vi "LHF.DB.Mongo.Collection.FindAndModify.vi"(6 "fields":refnum<k24>, 8 "error in (no error)":errorcluster, 9 "query":refnum<k24>, 10 "Collection":string, 11 "LHF.DB.Mongo in":refnum<class "LHF.DB.Mongo.lvclass">) -> (0 "error out":errorcluster, 2 "Document":string, 3 "LHF.DB.Mongo out":refnum<class "LHF.DB.Mongo.lvclass">, 5 "_id":string)   [LabVIEW 2013]
uses:
  LHF.DB.Mongo.lvclass
  C:/Users/Ricardo/Desktop/Projetos/LabVIEW-MongoDB/src/Driver/MongoDB.Driver.dll
  Driver/MongoDB.Driver.dll
  C:/Users/Ricardo/Desktop/Projetos/LabVIEW-MongoDB/src/Driver/MongoDB.Bson.dll
  Driver/MongoDB.Bson.dll
panel:
  in  "update":refnum<k24>
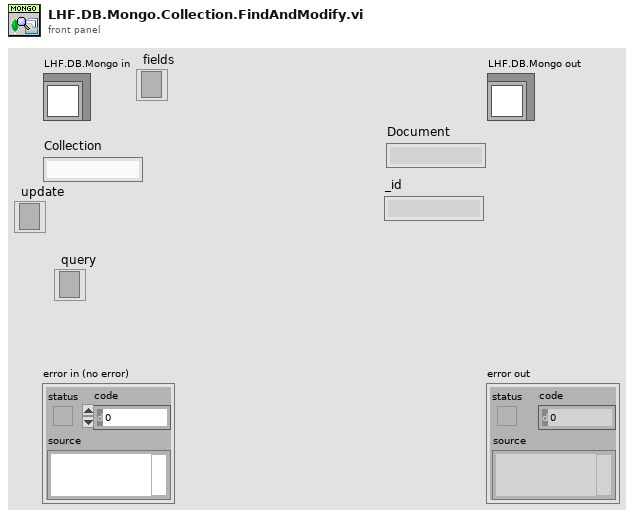
[diagram p1: front panel]
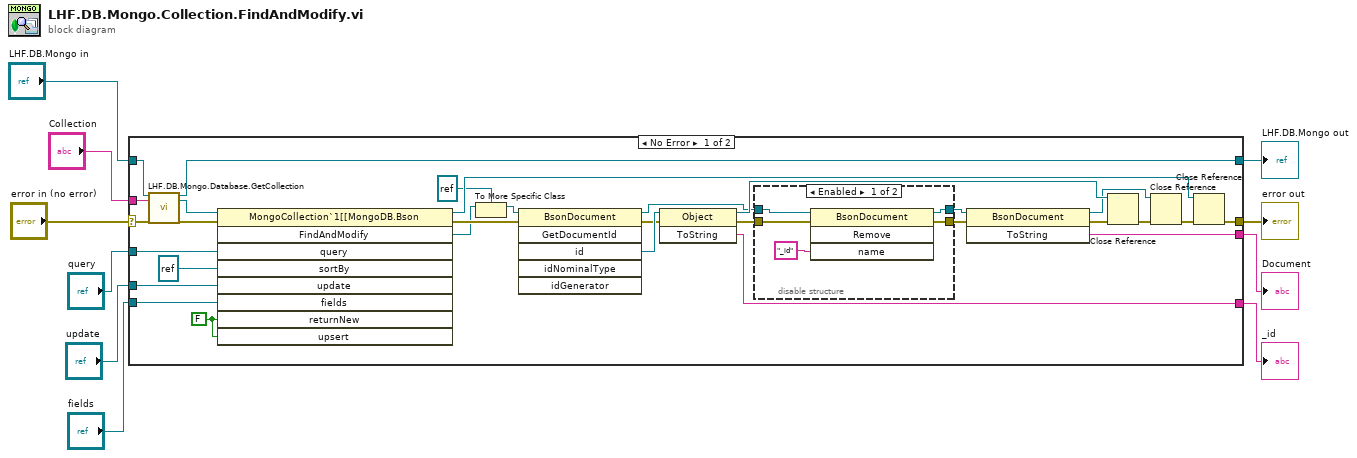
[diagram p0: block diagram]
diagram:
  n1 = case shown="No Error" "error in (no error)" {
    selector: "error in (no error)" -> [w34 w49]
    tunnel: [w36 w49] -> w9
    tunnel: [w39 w48] -> w7
    tunnel: "LHF.DB.Mongo in" -> [w38 w48]
    tunnel: "Collection" -> [w40 _]
    tunnel: "query" -> [w19 _]
    tunnel: [w21 _] -> w4
    tunnel: [w20 _] -> w3
    tunnel: "fields" -> [w12 _]
    tunnel: "update" -> [w11 _]
    frame No Error {
      w13 = FALSE ("returnNew")
      n2 = call "LHF.DB.Mongo.Database.GetCollection.vi"("LHF.DB.Mongo in"=w38, "collectionName"=w40, "error in (no error)"=w34) -> ("LHF.DB.Mongo in"=w39:refnum<class "LHF.DB.Mongo.lvclass">, "MongoCollection"=w35:refnum<k24>, "error out"=w33:errorcluster)  [unwired: 14 in]
      n3 = invoke class="MongoCollection`1[[MongoDB.Bson" method="FindAndModify"(reference=w35, error in=w33, "query"=w19, "sortBy"=refnum<k24> refnum, "update"=w11, "fields"=w12, "returnNew"=w13, "upsert"=w13) -> (reference out=w37:refnum<k24>, error out=w18:errorcluster, "FindAndModify"=w17:refnum<k24>)  [unwired: 1 in, 6 out]
      n4 = To More Specific Class(target class=refnum<k24> refnum ("BsonDocument"), reference=w17) -> (specific class reference=w16:refnum<k24>)  [unwired: 1 in, 1 out]
      n5 = invoke class="BsonDocument" method="GetDocumentId"(reference=w16, error in=w18) -> (reference out=w26:refnum<k24>, error out=w31:errorcluster, "id"=w32:refnum<k24>)  [unwired: 4 in, 3 out]
      n6 = invoke class="Object" method="ToString"(reference=w32, error in=w31) -> (reference out=w29:refnum<k24>, error out=w27:errorcluster, "ToString"=w21:string)  [unwired: 1 in]
      n7 = disable-structure shown="Enabled" {
        disable-tunnel: [w44 w47] -> w28
        disable-tunnel: w27 -> [w43 w46]
        disable-tunnel: w26 -> [w42 w47]
        disable-tunnel: [w41 w46] -> w23
        frame Enabled {
          n8 = invoke class="BsonDocument" method="Remove"(reference=w42, error in=w43, "name"="_id") -> (reference out=w44:refnum<k24>, error out=w41:errorcluster)  [unwired: 1 in, 2 out]
        }
        frame Disabled {
        }
      }
      n9 = invoke class="BsonDocument" method="ToString"(reference=w28, error in=w23) -> (reference out=w25:refnum<k24>, error out=w24:errorcluster, "ToString"=w20:string)  [unwired: 1 in]
      n10 = Close Reference(reference=w29, error in (no error)=w24) -> (error out=w30:errorcluster)
      n11 = Close Reference(reference=w25, error in (no error)=w30) -> (error out=w22:errorcluster)
      n12 = Close Reference(reference=w37, error in (no error)=w22) -> (error out=w36:errorcluster)
    }
    frame Error {
    }
  }
  "error out" <- w9
  "LHF.DB.Mongo out" <- w7
  "Document" <- w3
  "_id" <- w4
